vi "ISEG_HVBoard.ProcEvents.vi"(0 "i ref in":refnum<vi>, 5 "error in (no error)":errorcluster) -> (14 "i ref out":refnum<vi>, 19 "error out":errorcluster)   [LabVIEW 2014, in "ISEG_HVBoard.lvlib"]
doc: "This method is used to define the events the object will listen to. Add your own events here."
uses:
  ISEG_HVBoard.lvlib
  CSCore/BaseProcess/BaseProcess.event definition.ctl
  CSCore/CAEObj/CAEObj.event definition.ctl
  CSCore/BaseProcess/BaseProcess.descriptor string definition.ctl
  CSCore/BaseProcess/BaseProcess.lvlib
  CSCore/CAEObj/CAEObj.lvlib
panel:
  in  "event definition":T1={"CAEEvtDef"={"URL"="lvmsg://setKill", "enable"=TRUE, "ignoreResID"=FALSE}, "Data Descriptor"="S:1 n[Kill] //If Kill=True: Switch OFF at the max rate all system channels;"}
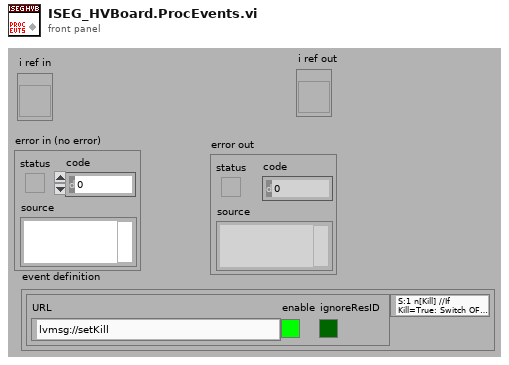
[diagram p1: front panel]
types:
  T1 = typedef "BaseProcess.lvlib/BaseProcess.event definition.ctl" = cluster{"CAEEvtDef":T2, "Data Descriptor":T3}
  T2 = typedef "CAEObj.lvlib/CAEObj.event definition.ctl" = cluster{"URL":string, "enable":bool, "ignoreResID":bool}
  T3 = typedef "BaseProcess.lvlib/BaseProcess.descriptor string definition.ctl" = string
  T4 = typedef "ISEG_HVBoard.lvlib/ISEG_HVBoard.i attribute.ctl" = cluster{"System Name":string, "Board ID":i32, "Prefix":string, "NrOfCh":cluster{"NrOfCh":i16, "DIM Status":T5}, "Status":cluster{"Status":i16, "DIM Status":T5}, "HardwareVLimit":cluster{"HVMax":dbl, "DIM Status":T5}, "BoardTemp":cluster{"Temp":dbl, "DIM Status":T5}, " Emcy":cluster{"Emcy":bool, "DIM Status":T5}}
  T5 = typedef "ISEG_HVBoard.lvlib/ISEG_HVBoard.DIM Status.ctl" = cluster{"no link":bool, "quality":i32, "Time Stamp":timestamp}
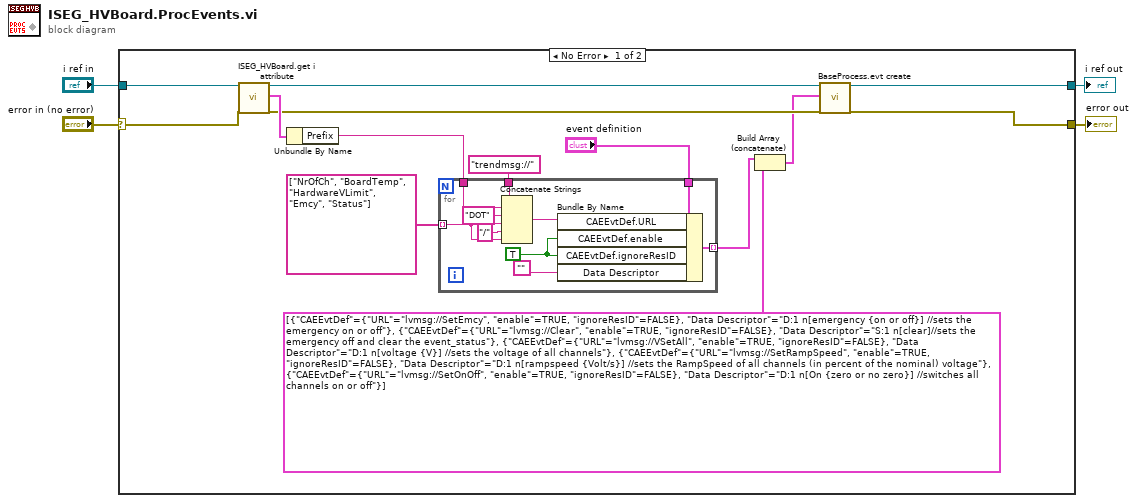
[diagram p0: block diagram]
diagram:
  n1 = case shown="No Error" "error in (no error)" {
    selector: "error in (no error)" -> [w5 w29]
    tunnel: "i ref in" -> [w12 w30]
    tunnel: [w11 w30] -> w3
    tunnel: [w10 w29] -> w2
    frame No Error {
      n2 = call "ISEG_HVBoard.get i attribute.vi"("i ref in"=w12, "error in (no error)"=w5) -> ("i ref out"=w14:refnum<vi>, "i attribute"=w16:T4, "error out"=w13:errorcluster)  [unwired: 15 in]
      n3 = Unbundle By Name(w16) -> ("Prefix"=w15:string)
      n4 = for {
        tunnel: "event definition" -> [w28]
        tunnel: "trendmsg://" -> [w27]
        tunnel: string[] ["NrOfCh", "BoardTemp", "HardwareVLimit", "Emcy", "Status"] -> [w22] mode=indexing
        tunnel: [w21] -> w8 mode=indexing
        tunnel: w15 -> [w19]
        w25 = TRUE ("CAEEvtDef.ignoreResID")
        n5 = Concatenate Strings(w27, w19, "DOT" ("string"), w22, "/" ("string"), w22) -> (w26:string)
        n6 = Bundle By Name(cluster=w28, "CAEEvtDef.URL"=w26, "CAEEvtDef.enable"=w25, "CAEEvtDef.ignoreResID"=w25, "Data Descriptor"="") -> (w21:T1)
      }
      n7 = Build Array (concatenate)(w8, T1[] [{"CAEEvtDef"={"URL"="lvmsg://SetEmcy", "enable"=TRUE, "ignoreResID"=FALSE}, "Data Descriptor"="D:1 n[emergency {on or off}] //sets the emergency on or off"}, {"CAEEvtDef"={"URL"="lvmsg://Clear", "enable"=TRUE, "ignoreResID"=FALSE}, "Data Descriptor"="S:1 n[clear]//sets the emergency off and clear the event_status"}, {"CAEEvtDef"={"URL"="lvmsg://VSetAll", "enable"=TRUE, "ignoreResID"=FALSE}, "Data Descriptor"="D:1 n[voltage {V}] //sets the voltage of all channels"}, {"CAEEvtDef"={"URL"="lvmsg://SetRampSpeed", "enable"=TRUE, "ignoreResID"=FALSE}, "Data Descriptor"="D:1 n[rampspeed {Volt/s}] //sets the RampSpeed of all channels (in percent of the nominal) voltage"}, {"CAEEvtDef"={"URL"="lvmsg://SetOnOff", "enable"=TRUE, "ignoreResID"=FALSE}, "Data Descriptor"="D:1 n[On {zero or no zero}] //switches all channels on or off"}]) -> (w7:T1[])
      n8 = call "BaseProcess.evt create.vi"("i ref in"=w14, "newEvents"=w7, "error in (no error)"=w13) -> ("i ref out"=w11:refnum<vi>, "error out"=w10:errorcluster)  [unwired: 13 in, 2 out]
    }
    frame Error {
    }
  }
  "i ref out" <- w3
  "error out" <- w2
